vi "BinaryReader.vi"() -> ()   [LabVIEW 2013]
uses:
  Files/Signal_Segment.ctl
  ControlDef/ProcessingMode.ctl
  BinaryReader_Params.ctl
  BinaryRead_State.ctl
  BinaryViewer_Params.ctl
  ReaderUpperLevelRefs.ctl
  _FileFormatConversion/UIC-DepthProfileFormat/DepthProfileFormat_Spectrum.ctl
  DepthProfile_Params.ctl
  _FileFormatConversion/UIC-DepthProfileFormat/LayerAverage_Params.ctl
  <vilib>/Analysis/baseanly.llb/Mean (DBL).vi
  <vilib>/Analysis/NI_AALBase.lvlib
panel:
  out "Comment":string
  in  "Open":bool caption="Quit"
  in  "Average":i32=1 min=1 step=1
  in  "nth layer":i32=1 min=1 step=1
  in  "Load All":bool caption="Quit"
  in  "width (Da)":dbl=0.5
  in  "m/z (Da)":dbl=12.0
  in  "Average#":i32=1 min=1 step=1
  out "Percentage":dbl(slide) scale=0.0..100.0 scale format="%.1f"
  out "Header":T1
  out "Spectrum":cluster{"mzArray":dbl[], "Spectrum":dbl[]}(graph)
  in  "Index":i32=1 min=0 step=1
  in  "Read_i":bool caption="Quit"
  in  "Indexing":bool caption="Quit"
  out "Signal+":T3={"SampleRate"=-1.0, "TrigDelay"=0.0, "SpecLength"=0.0, "DAQ_Range"=0.0, "Average#"=0, "Position"=[], "Spectrum"=[], "Calibr."=[], "Pressure"=-1.0, "Desp_LaserEnergy"=-1.0, "PI_LaserEnergy"=-1.0, "Voltages Table"=[], "ProcMode"=enum."None", "Threshold"=-1.0, "Comment"="", "TickCount"=0.0, "Time Stamp"=timestamp(0 s since 1904-01-01)} {"TickCount" format="%#.2f"}
  in  "Binary File Path":path
  in  "ForceQuit":bool caption="Quit"
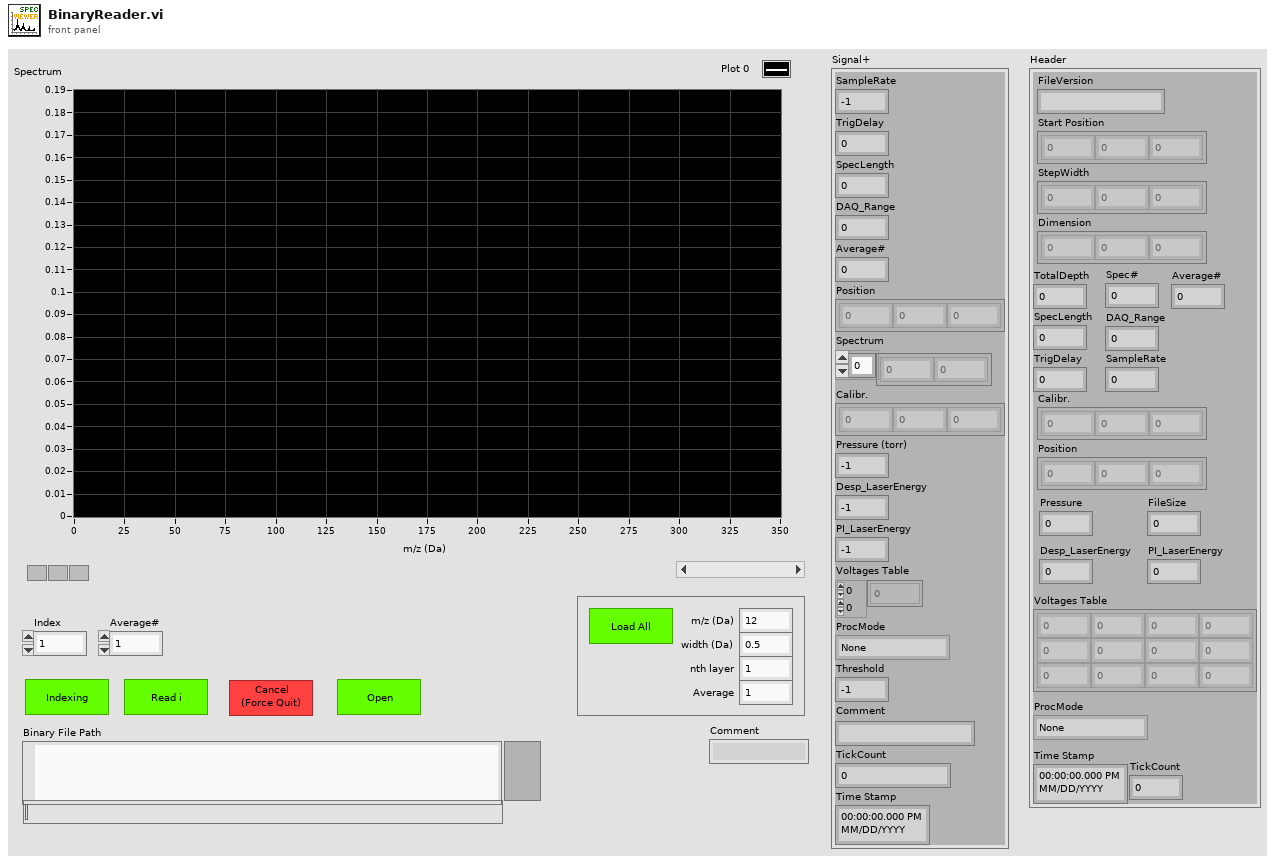
[diagram p1: front panel]
types:
  T1 = typedef "BinaryReader_Params.ctl" = cluster{"FileVersion":string, "Start Position":dbl[], "StepWidth":dbl[], "Dimension":i32[], "TotalDepth":i32, "Spec#":u32, "FileSize":i64, "Calibr.":dbl[], "Position":dbl[], "Pressure":dbl, "Desp_LaserEnergy":dbl, "PI_LaserEnergy":dbl, "SpecLength":dbl, "Average#":i32, "SampleRate":dbl, "DAQ_Range":dbl, "Voltages Table":sgl[][], "ProcMode":T2, "Time Stamp":timestamp, "TrigDelay":dbl, "TickCount":dbl}
  T2 = typedef "ProcessingMode.ctl" = enum16{"None", "Drop by Threshold", "TDC Simulate", "SetFilter"}
  T3 = typedef "Signal_Segment.ctl" = cluster{"SampleRate":dbl, "TrigDelay":dbl, "SpecLength":dbl, "DAQ_Range":dbl, "Average#":i32, "Position":dbl[], "Spectrum":sgl[], "Calibr.":dbl[], "Pressure":dbl, "Desp_LaserEnergy":dbl, "PI_LaserEnergy":dbl, "Voltages Table":sgl[][], "ProcMode":T2, "Threshold":dbl, "Comment":string, "TickCount":dbl, "Time Stamp":timestamp}
  T4 = typedef "ReaderUpperLevelRefs.ctl" = cluster{"Percentage":refnum<vi>, "ForceQuit":refnum<vi>, "Header":refnum<vi>}
  T5 = typedef "DepthProfileFormat_Spectrum.ctl" = cluster{"Average#":i16, "SpecLength":i32, "Spectrum":sgl[], "Cali.":dbl[], "Sample Rate":dbl}
  T6 = typedef "BinaryViewer_Params.ctl" = cluster{"State":enum16{"DisplaySingle", "DisplayMultiple", "LoadAll", "LayersAverage", "DepthProfile", "Clear"}, "Params.":variant}
  T7 = typedef "BinaryRead_State.ctl" = cluster{"State":enum16{"Open", "GetHeader", "Index", "Read_i", "Read_all", "Close", "Quit"}, "Params":variant}
  T8 = typedef "DepthProfile_Params.ctl" = cluster{"m/z":dbl, "width":dbl}
  T9 = typedef "LayerAverage_Params.ctl" = cluster{"Index+1":i32, "Average#":i32}
  T10 = enum16{"DisplaySingle", "DisplayMultiple", "LoadAll", "LayersAverage", "DepthProfile", "Clear"}
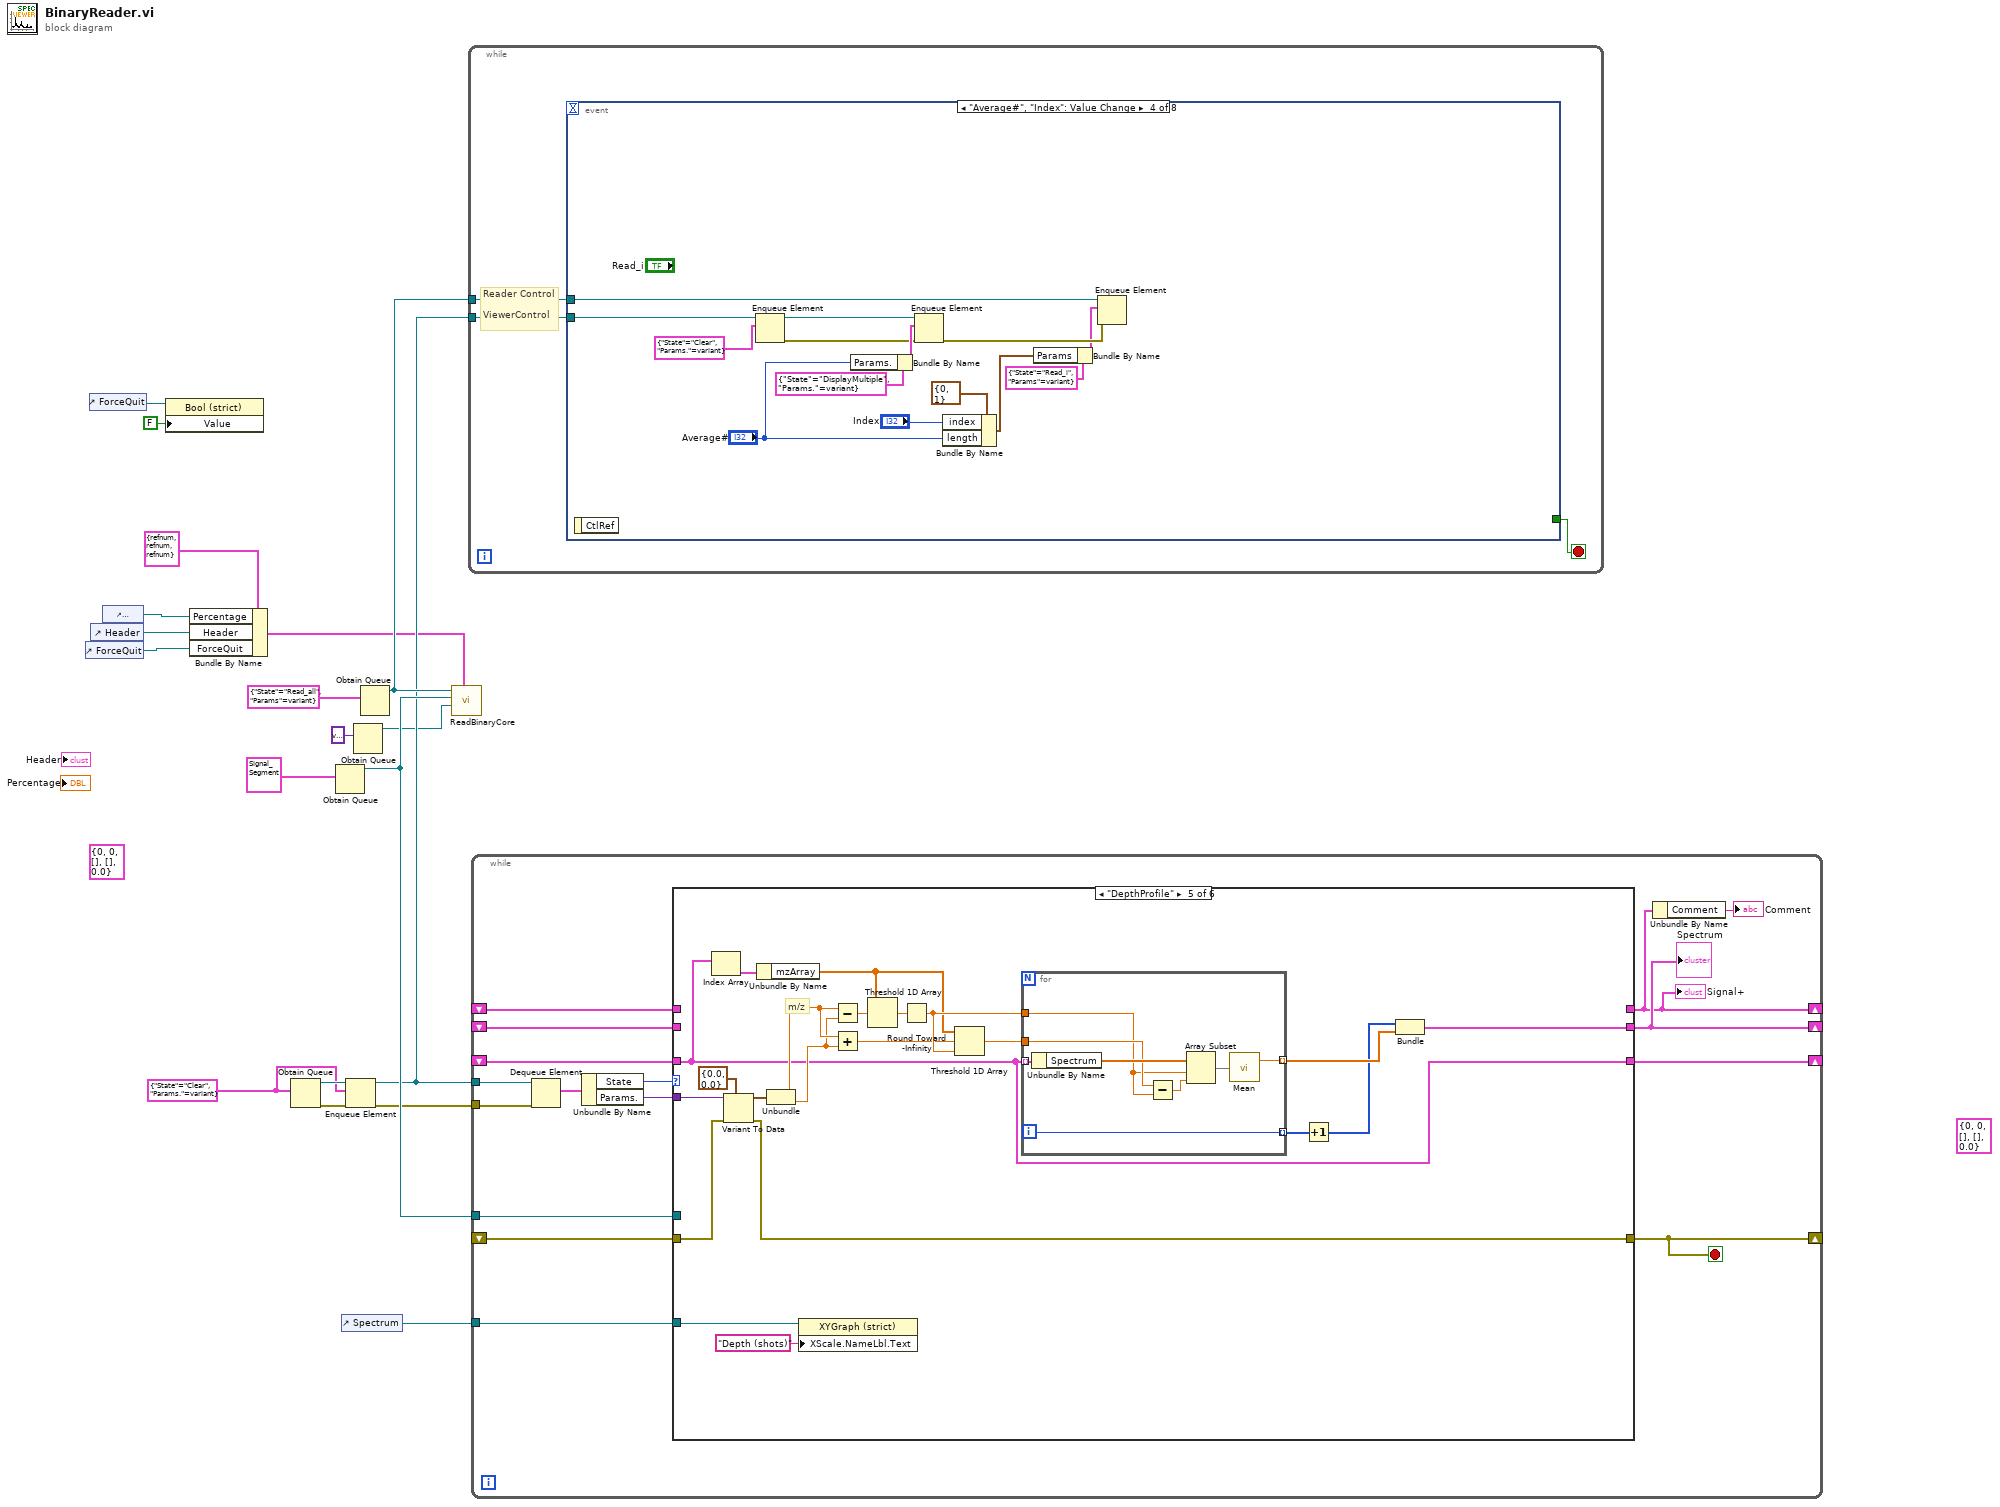
[diagram p0: block diagram]
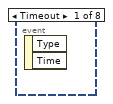
[diagram p2: hidden frame]
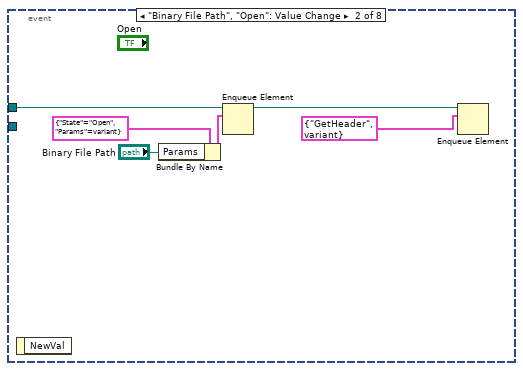
[diagram p3: hidden frame]
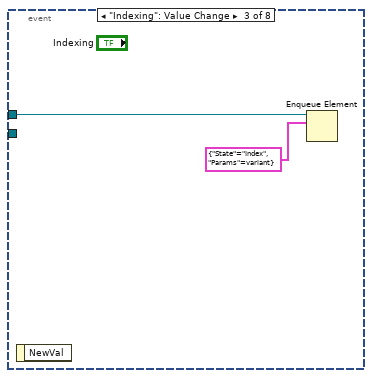
[diagram p4: hidden frame]
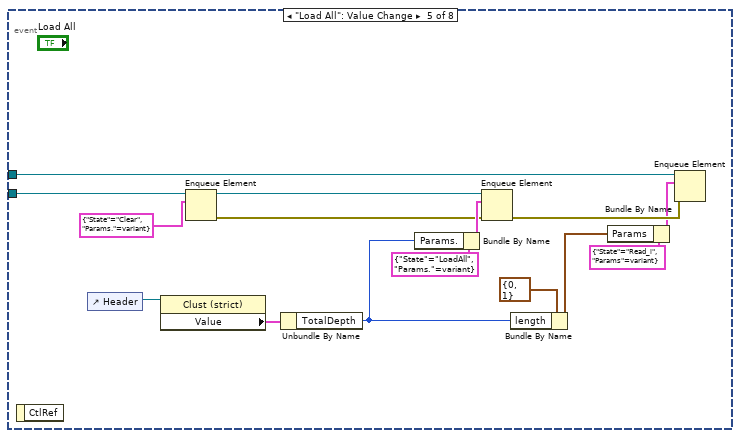
[diagram p5: hidden frame]
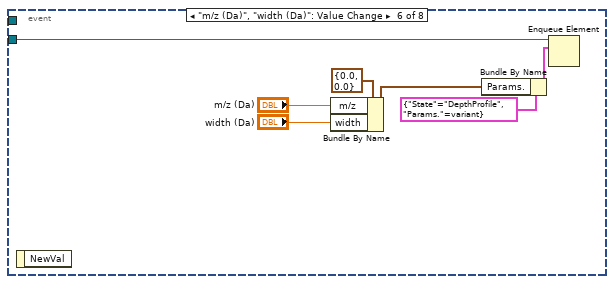
[diagram p6: hidden frame]
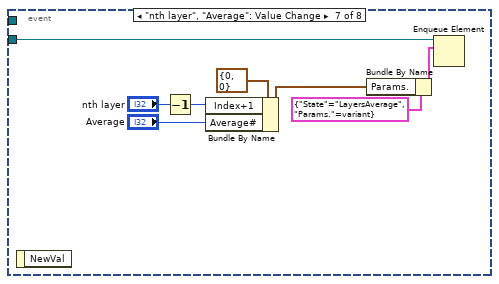
[diagram p7: hidden frame]
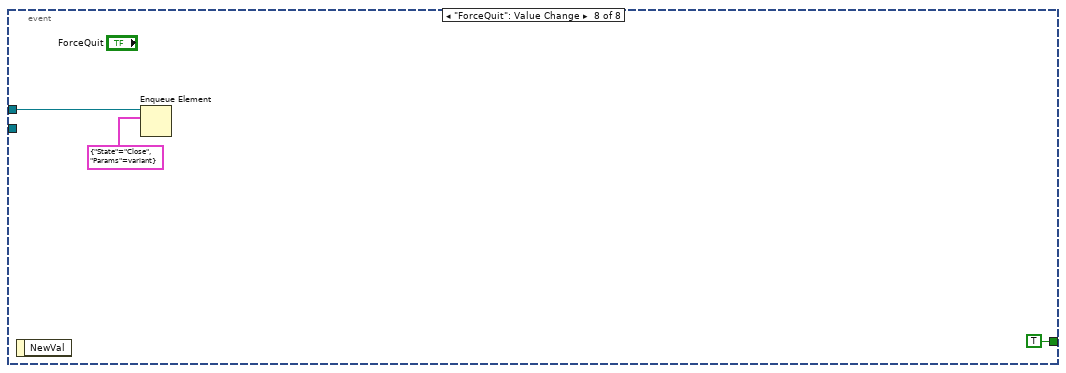
[diagram p8: hidden frame]
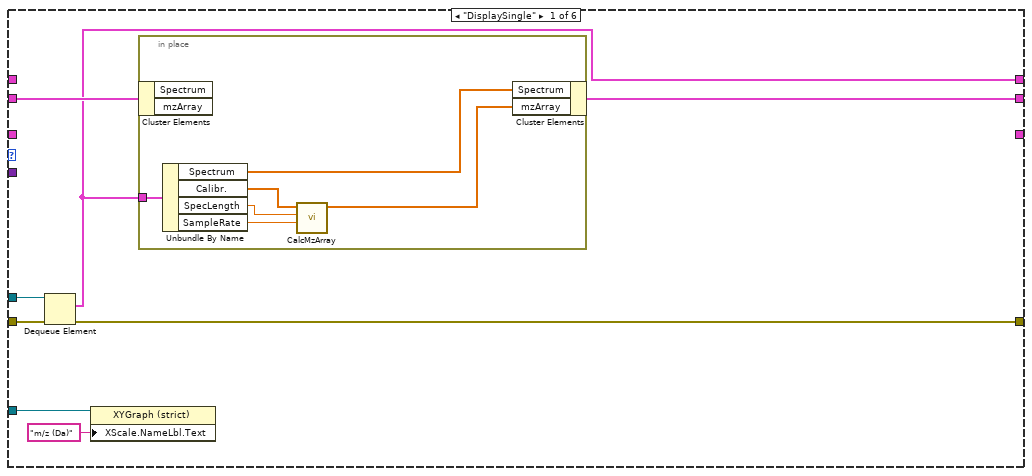
[diagram p9: hidden frame]
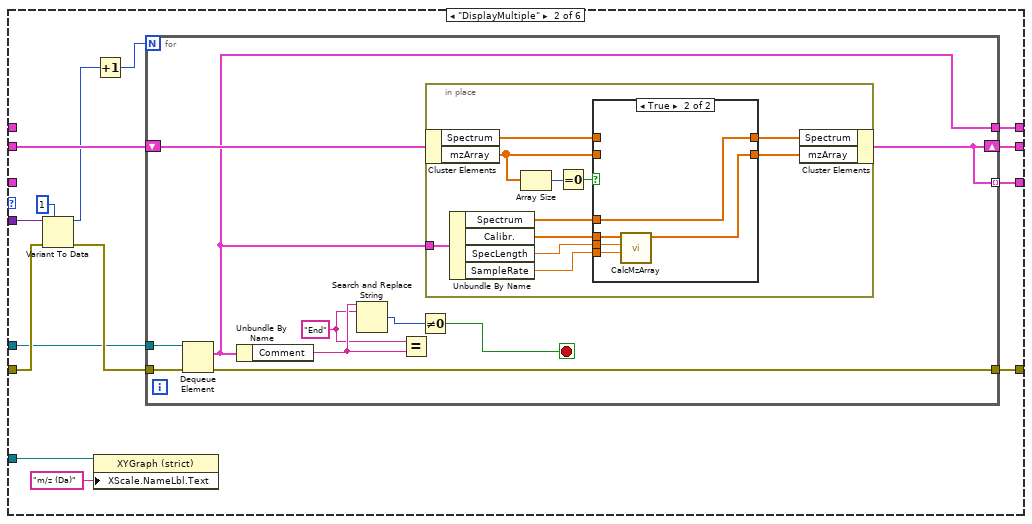
[diagram p10: hidden frame]
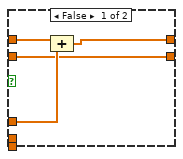
[diagram p11: hidden frame]
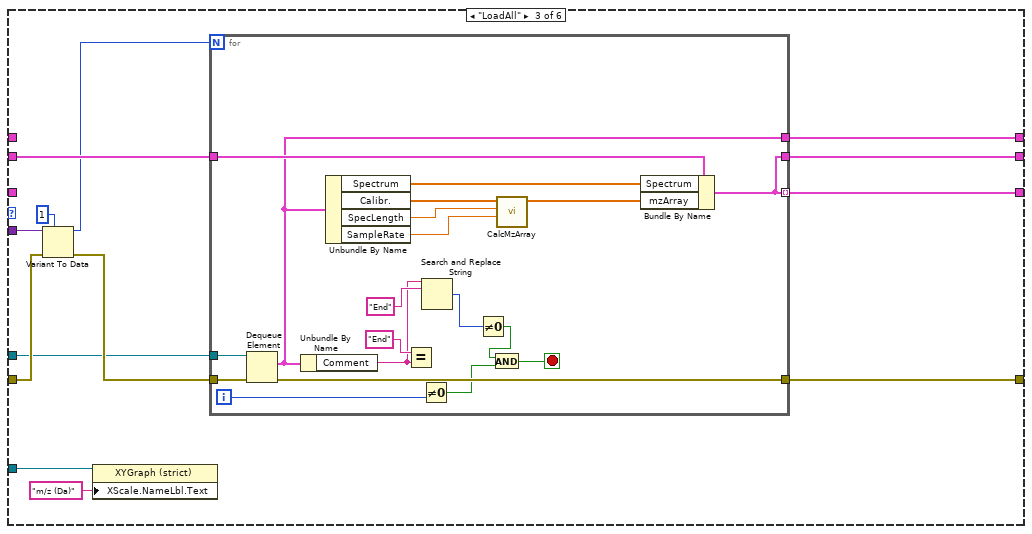
[diagram p12: hidden frame]
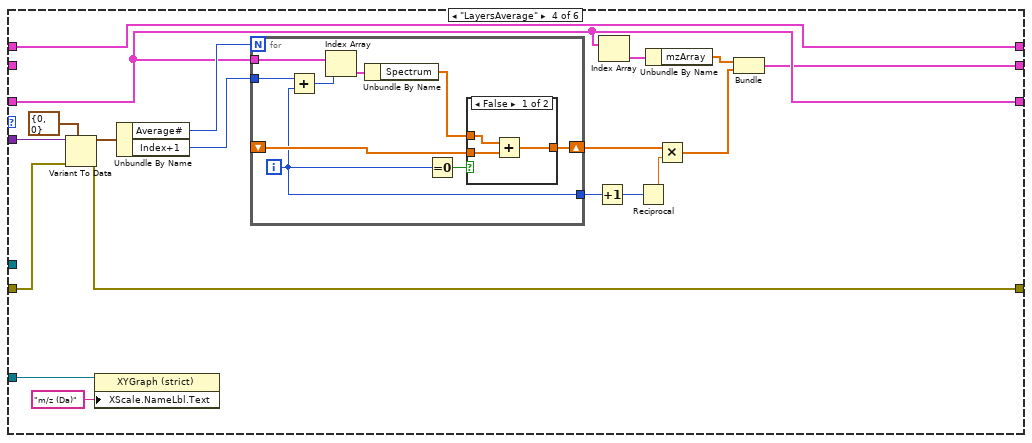
[diagram p13: hidden frame]
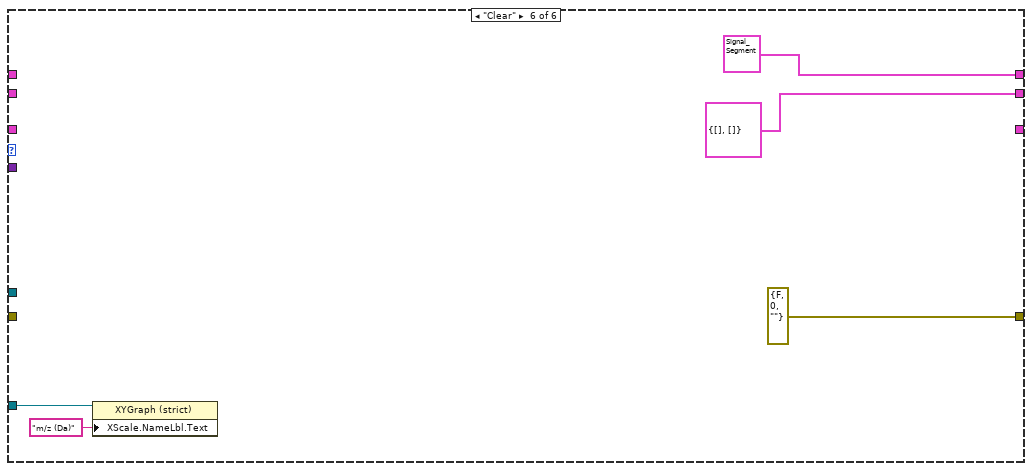
[diagram p15: hidden frame]
diagram:
  (unwired) T5 {"Average#"=0, "SpecLength"=0, "Spectrum"=[], "Cali."=[], "Sample Rate"=0.0} ("cluster")
  w12 = T6 {"State"=enum."Clear", "Params."=variant}
  (unwired) T5 {"Average#"=0, "SpecLength"=0, "Spectrum"=[], "Cali."=[], "Sample Rate"=0.0} ("cluster")
  n1 = control-ref of="ForceQuit"() -> (w6:refnum<vi>)
  n2 = control-ref of="ForceQuit"() -> (w15:refnum<vi>)
  n3 = control-ref of="Header"() -> (w3:refnum<vi>)
  n4 = control-ref of="Percentage"() -> (w7:refnum<vi>)
  n5 = property class="Bool (strict)"(reference=w15, "Value"=FALSE) -> ()  [unwired: 1 in, 2 out]
  n6 = Bundle By Name(cluster=T4 {"Percentage"=refnum, "ForceQuit"=refnum, "Header"=refnum}, "Percentage"=w7, "Header"=w3, "ForceQuit"=w6) -> (w4:T4)
  n7 = Obtain Queue(element data type=w12) -> (queue out=w13:refnum<queue>, error out=w11:errorcluster)  [unwired: 4 in, 1 out]
  n8 = Obtain Queue(element data type=T3 {"SampleRate"=0.0, "TrigDelay"=0.0, "SpecLength"=0.0, "DAQ_Range"=0.0, "Average#"=0, "Position"=[], "Spectrum"=[], "Calibr."=[], "Pressure"=0.0, "Desp_LaserEnergy"=0.0, "PI_LaserEnergy"=0.0, "Voltages Table"=[], "ProcMode"=enum."None", "Threshold"=0.0, "Comment"="", "TickCount"=0.0, "Time Stamp"=timestamp(0 s since 1904-01-01)} ("Signal Segment")) -> (queue out=w18:refnum<queue>)  [unwired: 4 in, 2 out]
  n9 = control-ref of="Spectrum"() -> (w8:refnum<vi>)
  n10 = Enqueue Element(queue=w13, element=w12, error in (no error)=w11) -> (queue out=w9:refnum<queue>, error out=w10:errorcluster)  [unwired: 1 in, 1 out]
  n11 = Obtain Queue(element data type=variant) -> (queue out=w2:refnum<queue>)  [unwired: 4 in, 2 out]
  n12 = Obtain Queue(element data type=T7 {"State"=enum."Read_all", "Params"=variant}) -> (queue out=w17:refnum<queue>)  [unwired: 4 in, 2 out]
  n13 = call "ReadBinaryCore.vi"("UpperLevelControlRefs."=w4, "metadata in"=w2, "data out in"=w18, "Control Queue in"=w17) -> ()  [unwired: 8 in]
  n14 = while {
    tunnel: w17 -> [w22]
    tunnel: w9 -> [w20]
    stop <- w21 stop-if-true
    # "Reader Control\n\nViewerControl"
    n15 = event shown="[3] \"Average#\", \"Index\": Value Change" {
      selector: _ -> [_ _ _ _ _ _ _ _]
      dyn-events: _ -> [_ _ _ _ _ _ _ _]
      timeout: _ -> [_ _ _ _ _ _ _ _]
      tunnel: w22 -> [_ w28 w29 w44 w59 _ _ w76]
      tunnel: [_ _ _ _ _ _ _ TRUE] -> w21
      tunnel: w20 -> [_ _ _ w43 w58 w63 w71 _]
      event Timeout {
        n16 = event-data() -> ()  [unwired: 1 in, 2 out]
      }
      event "Binary File Path", "Open": Value Change {
        n17 = event-data() -> ()  [unwired: 1 in, 1 out]
        n18 = Bundle By Name(cluster=T7 {"State"=enum."Open", "Params"=variant} ("element"), "Params"="Binary File Path") -> (w26:T7)
        n19 = Enqueue Element(queue=w28, element=w26) -> (queue out=w24:refnum<queue>)  [unwired: 2 in, 2 out]
        n20 = Enqueue Element(queue=w24, element=T7 {"State"=enum."GetHeader", "Params"=variant}) -> ()  [unwired: 2 in, 3 out]
      }
      event "Indexing": Value Change {
        n21 = event-data() -> ()  [unwired: 1 in, 1 out]
        n22 = Enqueue Element(queue=w29, element=T7 {"State"=enum."Index", "Params"=variant}) -> ()  [unwired: 2 in, 3 out]
      }
      event "Average#", "Index": Value Change {
        n23 = event-data() -> ()  [unwired: 1 in, 1 out]
        n24 = Enqueue Element(queue=w43, element=T6 {"State"=enum."Clear", "Params."=variant}) -> (queue out=w41:refnum<queue>, error out=w38:errorcluster)  [unwired: 2 in, 1 out]
        n25 = Bundle By Name(cluster=T6 {"State"=enum."DisplayMultiple", "Params."=variant} ("element"), "Params."="Average#") -> (w39:T6)
        n26 = Enqueue Element(queue=w41, element=w39, error in (no error)=w38) -> (error out=w37:errorcluster)  [unwired: 1 in, 2 out]
        n27 = Bundle By Name(cluster=cluster{"index":i32, "length":i32} {"index"=0, "length"=1}, "index"="Index", "length"="Average#") -> (w33:cluster{"index":i32, "length":i32})
        n28 = Bundle By Name(cluster=T7 {"State"=enum."Read_i", "Params"=variant} ("element"), "Params"=w33) -> (w35:T7)
        n29 = Enqueue Element(queue=w44, element=w35, error in (no error)=w37) -> ()  [unwired: 1 in, 3 out]
      }
      event "Load All": Value Change {
        n30 = event-data() -> ()  [unwired: 1 in, 1 out]
        n31 = control-ref of="Header"() -> (w47:refnum<vi>)
        n32 = property class="Clust (strict)"(reference=w47) -> ("Value"=w46:T1)  [unwired: 1 in, 2 out]
        n33 = Enqueue Element(queue=w58, element=T6 {"State"=enum."Clear", "Params."=variant}) -> (queue out=w56:refnum<queue>, error out=w53:errorcluster)  [unwired: 2 in, 1 out]
        n34 = Unbundle By Name(w46) -> ("TotalDepth"=w45:i32)
        n35 = Bundle By Name(cluster=T6 {"State"=enum."LoadAll", "Params."=variant} ("element"), "Params."=w45) -> (w54:T6)
        n36 = Enqueue Element(queue=w56, element=w54, error in (no error)=w53) -> (error out=w52:errorcluster)  [unwired: 1 in, 2 out]
        n37 = Bundle By Name(cluster=cluster{"index":i32, "length":i32} {"index"=0, "length"=1}, "length"=w45) -> (w48:cluster{"index":i32, "length":i32})
        n38 = Bundle By Name(cluster=T7 {"State"=enum."Read_i", "Params"=variant} ("element"), "Params"=w48) -> (w50:T7)
        n39 = Enqueue Element(queue=w59, element=w50, error in (no error)=w52) -> ()  [unwired: 1 in, 3 out]
      }
      event "m/z (Da)", "width (Da)": Value Change {
        n40 = event-data() -> ()  [unwired: 1 in, 1 out]
        n41 = Bundle By Name(cluster=T8 {"m/z"=0.0, "width"=0.0}, "m/z"="m/z (Da)", "width"="width (Da)") -> (w62:T8)
        n42 = Bundle By Name(cluster=T6 {"State"=enum."DepthProfile", "Params."=variant} ("element"), "Params."=w62) -> (w65:T6)
        n43 = Enqueue Element(queue=w63, element=w65) -> ()  [unwired: 2 in, 3 out]
      }
      event "nth layer", "Average": Value Change {
        n44 = event-data() -> ()  [unwired: 1 in, 1 out]
        n45 = Decrement(x="nth layer") -> (x-1=w67:i32)
        n46 = Bundle By Name(cluster=T9 {"Index+1"=0, "Average#"=0}, "Index+1"=w67, "Average#"="Average") -> (w70:T9)
        n47 = Bundle By Name(cluster=T6 {"State"=enum."LayersAverage", "Params."=variant} ("element"), "Params."=w70) -> (w73:T6)
        n48 = Enqueue Element(queue=w71, element=w73) -> ()  [unwired: 2 in, 3 out]
      }
      event "ForceQuit": Value Change {
        n49 = event-data() -> ()  [unwired: 1 in, 1 out]
        n50 = Enqueue Element(queue=w76, element=T7 {"State"=enum."Close", "Params"=variant}) -> ()  [unwired: 2 in, 3 out]
      }
    }
  }
  n51 = while {
    tunnel: w18 -> [w93]
    tunnel: w9 -> [w92]
    tunnel: w10 -> [w91]
    shift-right: [w87] -> _
    shift-left: _ -> [w88]
    shift-right: [w79] -> _
    shift-left: _ -> [w81]
    shift-right: [w85] -> _
    shift-left: _ -> [w84]
    shift-right: [w83] -> _
    shift-left: _ -> [w82]
    tunnel: w8 -> [w80]
    stop <- w85 stop-if-true
    n52 = Dequeue Element(queue=w92, error in (no error)=w91) -> (element=w90:T6)  [unwired: 1 in, 3 out]
    n53 = Unbundle By Name(w90) -> ("State"=w89:T10, "Params."=w86:variant)
    n54 = case shown="\"DepthProfile\"" w89 {
      tunnel: w93 -> [w101 w113 w155 _ _ _]
      tunnel: [w100 w121 w164 w196 w223 errorcluster {"status"=FALSE, "code"=0, "source"=""} ("error out")] -> w85
      tunnel: [w97 w118 w161 w185 w231 cluster{"mzArray":dbl[], "Spectrum":sgl[]} {"mzArray"=[], "Spectrum"=[]} ("Spectrum")] -> w87
      tunnel: w88 -> [w99 w120 w163 _ _ _]
      tunnel: [w98 w119 w162 w184 _ T3 {"SampleRate"=0.0, "TrigDelay"=0.0, "SpecLength"=0.0, "DAQ_Range"=0.0, "Average#"=0, "Position"=[], "Spectrum"=[], "Calibr."=[], "Pressure"=0.0, "Desp_LaserEnergy"=0.0, "PI_LaserEnergy"=0.0, "Voltages Table"=[], "ProcMode"=enum."None", "Threshold"=0.0, "Comment"="", "TickCount"=0.0, "Time Stamp"=timestamp(0 s since 1904-01-01)} ("Spectrum")] -> w79
      tunnel: w86 -> [_ w117 w160 w200 w229 _]
      tunnel: w84 -> [w96 w115 w157 w197 w224 _]
      tunnel: [_ w112 w154 w187 w218 _] -> w83
      tunnel: w82 -> [_ _ _ w187 w218 _]
      tunnel: w81 -> [_ _ _ w184 _ _]
      tunnel: w80 -> [w94 w110 w152 w201 w220 w245]
      frame "DisplaySingle" {
        n55 = Dequeue Element(queue=w101, error in (no error)=w96) -> (element=w98:T3, error out=w100:errorcluster)  [unwired: 1 in, 2 out]
        n56 = property class="XYGraph (strict)"(reference=w94, "XScale.NameLbl.Text"="m/z (Da)" ("X Scale.Name Label.Text")) -> ()  [unwired: 1 in, 2 out]
        n57 = in-place {
          in-place-border: w98 -> [w104]
          n58 = in-place-cluster #1(w99) -> ()  [unwired: 2 out]
          n59 = Unbundle By Name(w104) -> ("Spectrum"=w102:sgl[], "Calibr."=w105:dbl[], "SpecLength"=w106:dbl, "SampleRate"=w107:dbl)
          n60 = call "CalcMzArray.vi"("Sample Rate"=w107, "Depth"=w106, "mzCali. (a/b/c)"=w105) -> ("mzArray"=w103:dbl[])  [unwired: 8 in]
          n61 = in-place-cluster #1("Spectrum"=w102, "mzArray"=w103) -> (w97:cluster{"mzArray":dbl[], "Spectrum":dbl[]})
        }
      }
      frame "DisplayMultiple" {
        n62 = Variant To Data(error in=w115, type=1, Variant=w117) -> (data=w109:i32, error out=w114:errorcluster)
        n63 = property class="XYGraph (strict)"(reference=w110, "XScale.NameLbl.Text"="m/z (Da)" ("X Scale.Name Label.Text")) -> ()  [unwired: 1 in, 2 out]
        n64 = Increment(x=w109) -> (x+1=w108:i32)
        n65 = for {
          N: w108 -> [_]
          tunnel: w113 -> [w131]
          tunnel: [w130] -> w121
          tunnel: [w127] -> w119
          tunnel: w114 -> [w128]
          tunnel: [w126] -> w112 mode=indexing
          shift-right: [w126] -> w118
          shift-left: w120 -> [w129]
          stop <- w122 stop-if-true
          w124 = "End" ("x")
          n66 = Dequeue Element(queue=w131, error in (no error)=w128) -> (element=w127:T3, error out=w130:errorcluster)  [unwired: 1 in, 2 out]
          n67 = Unbundle By Name(w127) -> ("Comment"=w125:string)
          n68 = Search and Replace String(input string=w125, search string=w124) -> (number of replacements=w123:i32)  [unwired: 6 in, 3 out]
          n69 = Equal?(x=w124, y=w125) -> ()  [unwired: 1 out]
          n70 = Not Equal To 0?(x=w123) -> (x != 0?=w122:bool)
          n71 = in-place {
            in-place-border: w127 -> [w142]
            n72 = in-place-cluster #2(w129) -> ("Spectrum"=w140:dbl[], "mzArray"=w135:dbl[])
            n73 = Unbundle By Name(w142) -> ("Spectrum"=w138:sgl[], "Calibr."=w136:dbl[], "SpecLength"=w133:dbl, "SampleRate"=w132:dbl)
            n74 = Array Size(array=w135) -> (size(s)=w141:i32)
            n75 = Equal To 0?(x=w141) -> (x = 0?=w137:bool)
            n76 = case shown="True" w137 {
              tunnel: [w146 w147] -> w139
              tunnel: w138 -> [w145 w147]
              tunnel: w140 -> [w144 _]
              tunnel: w136 -> [_ w151]
              tunnel: w135 -> [w143 _]
              tunnel: [w143 w148] -> w134
              tunnel: w133 -> [_ w150]
              tunnel: w132 -> [_ w149]
              frame False {
                n77 = Compound Arithmetic op=ADD(w144, w145) -> (w146:dbl[])
              }
              frame True {
                n78 = call "CalcMzArray.vi"("Sample Rate"=w149, "Depth"=w150, "mzCali. (a/b/c)"=w151) -> ("mzArray"=w148:dbl[])  [unwired: 8 in]
              }
            }
            n79 = in-place-cluster #2("Spectrum"=w139, "mzArray"=w134) -> (w126:cluster{"mzArray":dbl[], "Spectrum":dbl[]})
          }
        }
      }
      frame "LoadAll" {
        n80 = Variant To Data(error in=w157, type=1, Variant=w160) -> (data=w158:i32, error out=w156:errorcluster)
        n81 = property class="XYGraph (strict)"(reference=w152, "XScale.NameLbl.Text"="m/z (Da)" ("X Scale.Name Label.Text")) -> ()  [unwired: 1 in, 2 out]
        n82 = for {
          N: w158 -> [_]
          tunnel: w155 -> [w183]
          tunnel: [w182] -> w164
          tunnel: w163 -> [w181]
          tunnel: [w175] -> w162
          tunnel: [w169] -> w161
          tunnel: w156 -> [w180]
          tunnel: [w169] -> w154 mode=indexing
          i -> [w176]
          stop <- w178 stop-if-true
          n83 = Dequeue Element(queue=w183, error in (no error)=w180) -> (element=w175:T3, error out=w182:errorcluster)  [unwired: 1 in, 2 out]
          n84 = Unbundle By Name(w175) -> ("Comment"=w167:string)
          n85 = Unbundle By Name(w175) -> ("Spectrum"=w174:sgl[], "Calibr."=w173:dbl[], "SpecLength"=w171:dbl, "SampleRate"=w170:dbl)
          n86 = Equal?(x="End", y=w167) -> ()  [unwired: 1 out]
          n87 = Not Equal To 0?(x=w176) -> (x != 0?=w177:bool)
          n88 = Search and Replace String(input string=w167, search string="End" ("x")) -> (number of replacements=w166:i32)  [unwired: 6 in, 3 out]
          n89 = Not Equal To 0?(x=w166) -> (x != 0?=w165:bool)
          n90 = And(x=w165, y=w177) -> (x .and. y?=w178:bool)
          n91 = call "CalcMzArray.vi"("Sample Rate"=w170, "Depth"=w171, "mzCali. (a/b/c)"=w173) -> ("mzArray"=w172:dbl[])  [unwired: 8 in]
          n92 = Bundle By Name(cluster=w181, "Spectrum"=w174, "mzArray"=w172) -> (w169:cluster{"mzArray":dbl[], "Spectrum":dbl[]})
        }
      }
      frame "LayersAverage" {
        n93 = Variant To Data(error in=w197, type=T9 {"Index+1"=0, "Average#"=0}, Variant=w200) -> (data=w198:T9, error out=w196:errorcluster)
        n94 = property class="XYGraph (strict)"(reference=w201, "XScale.NameLbl.Text"="m/z (Da)" ("X Scale.Name Label.Text")) -> ()  [unwired: 1 in, 2 out]
        n95 = Unbundle By Name(w198) -> ("Average#"=w189:i32, "Index+1"=w190:i32)
        n96 = for {
          N: w189 -> [_]
          tunnel: w187 -> [w211]
          tunnel: w190 -> [w209]
          shift-right: [w207] -> w195
          shift-left: _ -> [w206]
          tunnel: [w203] -> w192
          i -> [w203]
          n97 = Add(x=w209, y=w203) -> (x+y=w208:i32)
          n98 = Index Array(array=w211, index=w208) -> (element=w210:cluster{"mzArray":dbl[], "Spectrum":dbl[]})
          n99 = Unbundle By Name(w210) -> ("Spectrum"=w205:dbl[])
          n100 = Equal To 0?(x=w203) -> (x = 0?=w204:bool)
          n101 = case shown="False" w204 {
            tunnel: [w214 w215] -> w207
            tunnel: w206 -> [w213 _]
            tunnel: w205 -> [w212 w215]
            frame False {
              n102 = Add(x=w212, y=w213) -> (x+y=w214:dbl[])
            }
            frame True {
            }
          }
        }
        n103 = Increment(x=w192) -> (x+1=w191:i32)
        n104 = Index Array(array=w187) -> (element=w188:cluster{"mzArray":dbl[], "Spectrum":dbl[]})  [unwired: 1 in]
        n105 = Reciprocal(x=w191) -> (1/x=w193:dbl)
        n106 = Unbundle By Name(w188) -> ("mzArray"=w186:dbl[])
        n107 = Multiply(x=w195, y=w193) -> (x*y=w194:dbl[])
        n108 = Bundle("mzArray"=w186, w194) -> (w185:cluster{"mzArray":dbl[], dbl[]})  [unwired: 1 in]
      }
      frame "DepthProfile" {
        # "m/z"
        n109 = Index Array(array=w218) -> (element=w217:cluster{"mzArray":dbl[], "Spectrum":dbl[]})  [unwired: 1 in]
        n110 = Variant To Data(error in=w224, type=T8 {"m/z"=0.0, "width"=0.0}, Variant=w229) -> (data=w227:T8, error out=w223:errorcluster)
        n111 = Unbundle By Name(w217) -> ("mzArray"=w216:dbl[])
        n112 = Unbundle(w227) -> ("m/z"=w226:dbl, "width"=w225:dbl)
        n113 = property class="XYGraph (strict)"(reference=w220, "XScale.NameLbl.Text"="Depth (shots)" ("X Scale.Name Label.Text")) -> ()  [unwired: 1 in, 2 out]
        n114 = Subtract(x=w226, y=w225) -> (x-y=w233:dbl)
        n115 = Add(x=w226, y=w225) -> (x+y=w232:dbl)
        n116 = Threshold 1D Array(2:w233, 3:w216) -> (0:w236:dbl)  [unwired: 1 in]
        n117 = Round Toward -Infinity(1:w236) -> (0:w234:dbl)
        n118 = Threshold 1D Array(1:w234, 2:w232, 3:w216) -> (0:w235:dbl)
        n119 = for {
          tunnel: w218 -> [w244] mode=indexing
          tunnel: [w240] -> w230 mode=indexing
          tunnel: w235 -> [w239]
          tunnel: w234 -> [w238]
          tunnel: [w237] -> w222 mode=indexing
          i -> [w237]
          n120 = Unbundle By Name(w244) -> ("Spectrum"=w243:dbl[])
          n121 = Subtract(x=w239, y=w238) -> (x-y=w242:dbl)
          n122 = Array Subset(array=w243, index=w238, length=w242) -> (w241:dbl[])
          n123 = call-poly <vilib>:"Mean.vi"("X"=w241) -> ("mean"=w240:dbl)  [unwired: 1 out]
        }
        n124 = Increment(x=w222) -> (x+1=w221:i32[])
        n125 = Bundle(w221, w230) -> (w231:cluster{i32[], dbl[]})  [unwired: 1 in]
      }
      frame "Clear" {
        n126 = property class="XYGraph (strict)"(reference=w245, "XScale.NameLbl.Text"="m/z (Da)" ("X Scale.Name Label.Text")) -> ()  [unwired: 1 in, 2 out]
      }
    }
    "Spectrum" <- w87
    "Signal+" <- w79
    n127 = Unbundle By Name(w79) -> ("Comment"=→"Comment":string)
  }
